vi "String.Replace Variable Items.vi"(10 "Variable List":string[][](array[string]), 11 "String In":string="$Year_$Month_$Day") -> (3 "String Out":string)   [LabVIEW 2018]
panel:
  # "Name Value"
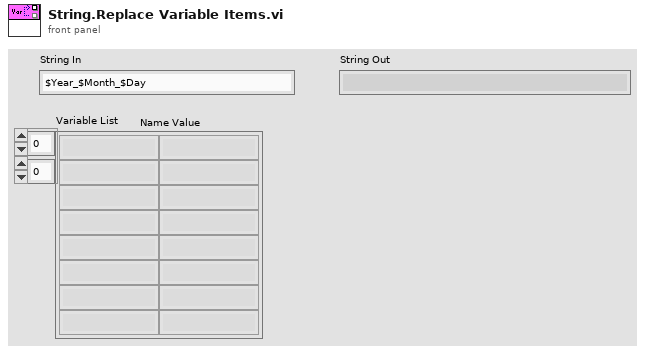
[diagram p1: front panel]
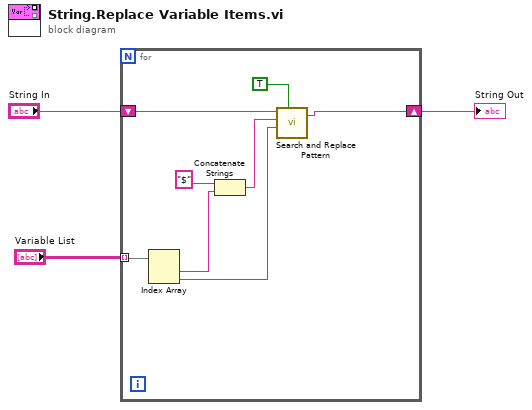
[diagram p0: block diagram]
diagram:
  n1 = for {
    tunnel: "Variable List" -> [w9] mode=indexing
    shift-right: [w5] -> w1
    shift-left: "String In" -> [w11]
    n2 = Index Array(array=w9) -> (element #1=w8:string, element #2=w6:string)  [unwired: 2 in]
    n3 = Concatenate Strings("$", w8) -> (w7:string)
    n4 = call <vilib>:"Search and Replace Pattern.vi"("string"=w11, "regular expression (\"\")"=w7, "replace string (\"\")"=w6, "replace all? (F)"=TRUE) -> ("result string"=w5:string)  [unwired: 1 in, 1 out]
  }
  "String Out" <- w1
